vi "get_batchID.vi"(2 "error in (no error)":errorcluster, 3 "UserID":string) -> (0 "error out":errorcluster, 1 "BatchID output":string[](array[string]))   [LabVIEW 2009]
uses:
  <vilib>/addons/database/Recordset.llb/Rec Destroy - Connection.vi
  <vilib>/addons/database/Recordset.llb/Rec Fetch Recordset Data (R).vi
  <vilib>/addons/database/Connection.llb/Conn Execute.vi
  <vilib>/addons/database/Connection.llb/DB Tools Open Connec (String).vi
  DB_Info.vi
  <vilib>/addons/database/_DB Variant To Data/Database Variant To Data.xnode
  <vilib>/addons/database/NI_Database_API.lvlib
panel:
  out "concatenated string":string
  out "BatchID Drop-down":string(combo)
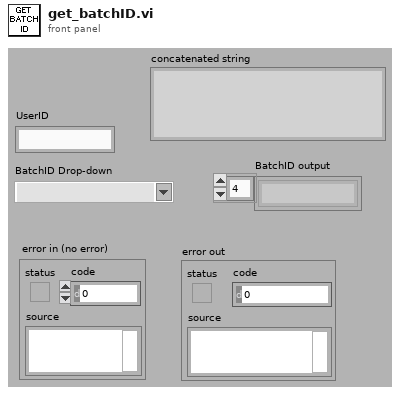
[diagram p1: front panel]
types:
  T1 = typedef "NI_Database_API.lvlib/Conn ObjectReference.ctl" = refnum<k1>
  T2 = typedef "NI_Database_API.lvlib/Rec ObjectReference.ctl" = refnum<k1>
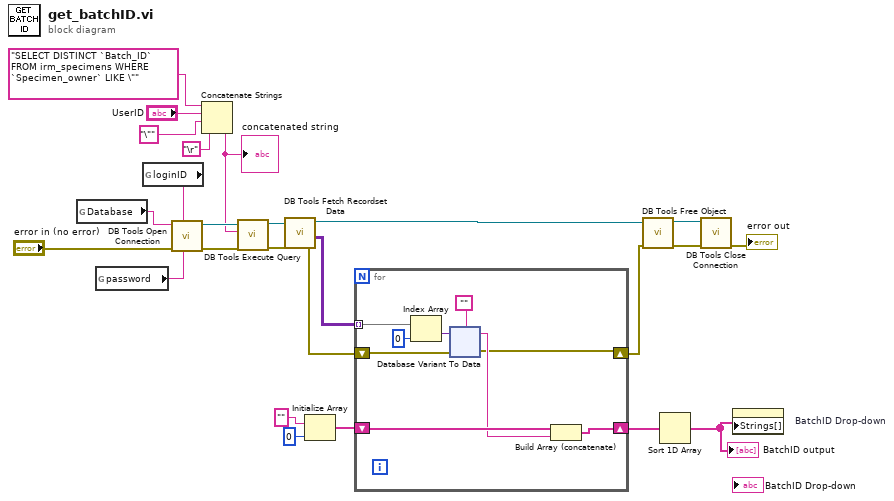
[diagram p0: block diagram]
diagram:
  n1 = global read "DB_Info.vi" "Database"() -> (w23:string)
  n2 = global read "DB_Info.vi" "password"() -> (w22:string)
  n3 = global read "DB_Info.vi" "loginID"() -> (w25:string)
  n4 = call-poly <vilib>:"DB Tools Open Connection.vi"("password"=w22, "userID"=w25, "error in (no error)"="error in (no error)", "connection information"=w23) -> ("error out"=w16:errorcluster, "connection reference"=w17:T1)  [unwired: 1 in, 3 out]
  n5 = Concatenate Strings("SELECT DISTINCT `Batch_ID` FROM irm_specimens WHERE  `Specimen_owner` LIKE \"", "UserID", "\"", "\r") -> (w12:string)
  "concatenated string" <- w12
  n6 = call-poly <vilib>:"DB Tools Execute Query.vi"("error in (no error)"=w16, "SQL query"=w12, "connection reference"=w17) -> ("error out"=w11:errorcluster, "recordset reference"=w10:T2)  [unwired: 5 in]
  n7 = call-poly <vilib>:"DB Tools Fetch Recordset Data.vi"("error in (no error)"=w11, "recordset reference"=w10) -> ("error out"=w5:errorcluster, "recordset data"=w7:variant[][], "recordset reference out"=w3:T2)  [unwired: 3 in]
  n8 = Initialize Array("" ("userID"), 0 ("dimension size")) -> (w19:string[])
  n9 = for {
    shift-right: [w27] -> w18
    shift-left: w19 -> [w29]
    tunnel: w7 -> [w30] mode=indexing
    shift-right: [w26] -> w4
    shift-left: w5 -> [w33]
    n10 = Index Array(array=w30, index=0 ("disabled index (col)")) -> (element=w34:variant)
    n11 = xnode "Database Variant To Data"("database variant"=w34, "error in"=w33, "type"="") -> ("data"=w28:string, "error out"=w26:errorcluster)
    n12 = Build Array (concatenate)(w29, w28) -> (w27:string[])
  }
  n13 = call-poly <vilib>:"DB Tools Free Object.vi"("error in (no error)"=w4, "recordset reference"=w3) -> ("error out"=w8:errorcluster, "connection reference"=w9:T1)  [unwired: 8 in]
  n14 = Sort 1D Array(array=w18) -> (sorted array=w6:string[])
  "BatchID output" <- w6
  n15 = call <vilib>:"DB Tools Close Connection.vi"("error in (no error)"=w8, "connection reference"=w9) -> ("error out"=→"error out":errorcluster)  [unwired: 5 out]
  n16 = property on="BatchID Drop-down" class="CmbBox"("Strings[]"=w6) -> ()  [unwired: 2 in, 2 out]
